vi "Adjust Dashboard Window Mod.vi"(6 "Sizing Refnums":T1, 7 "Stop?":bool, 9 "Size Constraints":cluster{"min tab width":i32, "w/h":dbl}, 10 "VI":refnum<vi>, 11 "Notifier in":refnum<notifier>) -> ()   [LabVIEW 2015]
uses:
  <vilib>/Utility/miscctls.llb/LVRectTypeDef.ctl
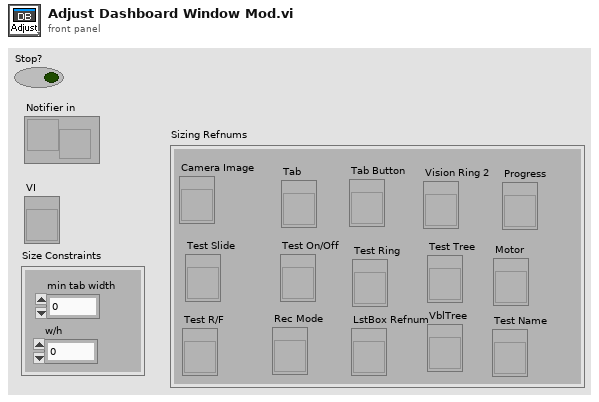
[diagram p1: front panel]
types:
  T1 = cluster{"Camera Image":refnum<vi>, "Tab":refnum<vi>, "Tab Button":refnum<vi>, "Vision Ring 2":refnum<vi>, "Rec Mode":refnum<vi>, "Test Slide":refnum<vi>, "Test On/Off":refnum<vi>, "Test Ring":refnum<vi>, "Test R/F":refnum<vi>, "Test Name":refnum<vi>, "Motor":refnum<vi>, "Progress":refnum<vi>, "LstBox Refnum":refnum<vi>, "Test Tree":refnum<vi>, "VblTree":refnum<vi>}
  T2 = typedef "LVRectTypeDef.ctl" = cluster{"Left":i16, "Top":i16, "Right":i16, "Bottom":i16}
  T3 = typedef "LVPointTypeDef.ctl" = cluster{"Horizontal":i16, "Vertical":i16}
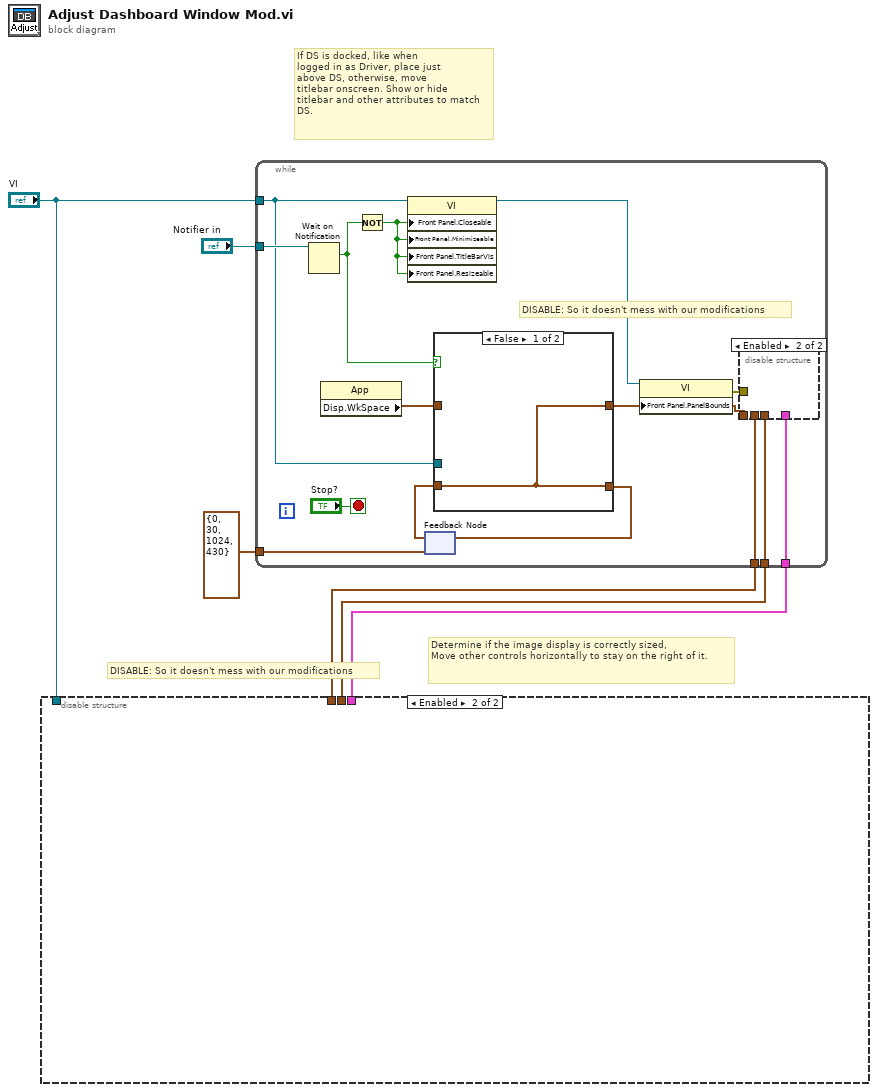
[diagram p0: block diagram]
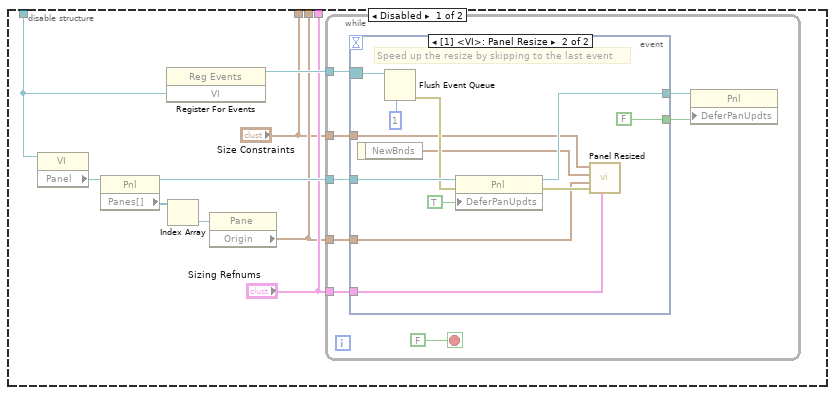
[diagram p2: hidden frame]
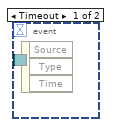
[diagram p3: hidden frame]
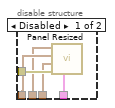
[diagram p4: hidden frame]
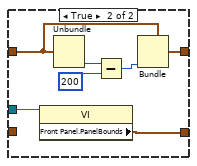
[diagram p5: hidden frame]
diagram:
  # "DISABLE: So it doesn't mess with our modifications"
  # "Determine if the image display is correctly sized,\nMove other controls horizontally to stay on the right of it."
  # "If DS is docked, like when\nlogged in as Driver, place just\nabove DS, otherwise, move\ntitlebar onscreen. Show or hide\ntitlebar and other attributes to match\nDS."
  n1 = disable-structure shown="Enabled" {
    disable-tunnel: "VI" -> [w14 _]
    disable-tunnel: ["Sizing Refnums" _] -> w4
    disable-tunnel: [w8 _] -> w3
    disable-tunnel: ["Size Constraints" _] -> w2
    frame Disabled {
      n2 = property class="VI"(reference=w14) -> ("Panel"=w13:refnum<vi>)  [unwired: 1 in, 2 out]
      n3 = property class="Pnl"(reference=w13) -> (reference out=w10:refnum<vi>, "Panes[]"=w12:refnum<vi>[])  [unwired: 1 in, 1 out]
      n4 = register-events(w14) -> (reference out=w15:refnum<event-registration>)  [unwired: 2 in, 1 out]
      n5 = Index Array(array=w12) -> (element=w11:refnum<vi>)  [unwired: 1 in]
      n6 = property class="Pane"(reference=w11) -> ("Origin"=w8:T3)  [unwired: 1 in, 2 out]
      n7 = while {
        tunnel: w15 -> [w22]
        tunnel: "Sizing Refnums" -> [w21]
        tunnel: "Size Constraints" -> [w20]
        tunnel: w8 -> [w19]
        tunnel: w10 -> [w18]
        stop <- FALSE stop-if-true
        n8 = event shown="[1] <VI>: Panel Resize" {
          selector: w22 -> [_ w32]
          dyn-events: _ -> [_ _]
          timeout: _ -> [_ _]
          tunnel: w21 -> [_ w24]
          tunnel: w20 -> [_ w27]
          tunnel: w19 -> [_ w25]
          tunnel: w18 -> [_ w35]
          tunnel: [_ FALSE ("Defer Panel Updates")] -> w17
          tunnel: [_ w29] -> w16
          event Timeout {
            n9 = event-data() -> ()  [unwired: 1 in, 3 out]
          }
          event Panel Resize {
            # "Speed up the resize by skipping to the last event"
            n10 = event-data() -> ("NewBnds"=w26:T2)  [unwired: 1 in]
            n11 = Flush Event Queue(0:w32, 5:1 ("keep most recent")) -> (11:w30:errorcluster)  [unwired: 4 in, 2 out]
            n12 = property class="Pnl"(reference=w35, error in=w30, "DeferPanUpdts"=TRUE ("Defer Panel Updates")) -> (reference out=w29:refnum<vi>, error out=w28:errorcluster)
            n13 = call "Panel Resized.vi"("Sizing Refnums"=w24, "error in (no error)"=w28, "Origin"=w25, "NewBnds"=w26, "Size Constraints"=w27) -> ()  [unwired: 6 in, 1 out]
          }
        }
        n14 = property class="Pnl"(reference=w16, "DeferPanUpdts"=w17) -> ()  [unwired: 1 in, 2 out]
      }
    }
    frame Enabled {
    }
  }
  n15 = while {
    tunnel: "Notifier in" -> [w49]
    tunnel: "VI" -> [w40]
    tunnel: w4 -> [w45]
    tunnel: w3 -> [w44]
    tunnel: w2 -> [w42]
    tunnel: T2 {"Left"=0, "Top"=30, "Right"=1024, "Bottom"=430} ("Front Panel.PanelBounds") -> [w37]
    stop <- "Stop?" stop-if-true
    # "DISABLE: So it doesn't mess with our modifications"
    n16 = Wait on Notification(notifier=w49) -> (notification=w41:bool)  [unwired: 3 in, 3 out]
    n17 = property class="App"() -> ("Disp.WkSpace"=w48:T2)  [unwired: 2 in, 2 out]
    n18 = Not(x=w41) -> (.not. x?=w36:bool)
    n19 = property class="VI"(reference=w40, "Front Panel.Closeable"=w36, "Front Panel.Minimizeable"=w36, "Front Panel.TitleBarVis"=w36, "Front Panel.Resizeable"=w36) -> (reference out=w47:refnum<vi>)  [unwired: 1 in, 1 out]
    n20 = feedback #1(w37) -> (w38:T2)
    n21 = case shown="False" w41 {
      tunnel: w48 -> [_ w59]
      tunnel: [w56 w60] -> w43
      tunnel: w40 -> [_ w58]
      tunnel: [w56 w57] -> w39
      tunnel: w38 -> [w56 _]
      frame False {
      }
      frame True {
        n22 = property class="VI"(reference=w58) -> ("Front Panel.PanelBounds"=w57:T2)  [unwired: 1 in, 2 out]
        n23 = Unbundle(w59) -> ("Bottom"=w63:i16)  [unwired: 3 out]
        n24 = Subtract(x=w63, y=200) -> (x-y=w61:i32)
        n25 = Bundle(cluster=w59, "Bottom"=w61) -> (w60:T2)  [unwired: 3 out]
      }
    }
    n26 = feedback-in #1(w39) -> ()
    n27 = property class="VI"(reference=w47, "Front Panel.PanelBounds"=w43) -> (error out=w46:errorcluster)  [unwired: 1 in, 1 out]
    n28 = disable-structure shown="Enabled" {
      disable-tunnel: w46 -> [w55 _]
      disable-tunnel: w45 -> [w54 _]
      disable-tunnel: w44 -> [w53 _]
      disable-tunnel: w43 -> [w52 _]
      disable-tunnel: w42 -> [w51 _]
      frame Disabled {
        n29 = call "Panel Resized.vi"("Sizing Refnums"=w54, "error in (no error)"=w55, "Origin"=w53, "NewBnds"=w52, "Size Constraints"=w51) -> ()  [unwired: 6 in, 1 out]
      }
      frame Enabled {
      }
    }
  }
